vi "Map Initialization Behaviour.vi"(11 "initialize and close session behavior in":T1) -> (3 "initialization_behavior":T2)   [LabVIEW 2021, in "Session Management niDAQmx.lvlib" / "Session Factory.lvclass"]
doc: "Maps the measurement plug-in initialization behavior enum with the gRPC DAQmx initialization behaviour enum."
uses:
  Session Factory.lvclass
  NI DAQmx Client/RPC Messages/nidevice_grpc_SessionInitializationBehavior.ctl
  <vilib>/Plug-In SDKs/Sessions/Instrument/ISession Factory/Initialize and Close Session Behavior.ctl
  NI DAQmx Client/NI_DAQmx_client.lvlib
  <vilib>/Plug-In SDKs/Sessions/Instrument/ISession Factory/ISession Factory.lvclass
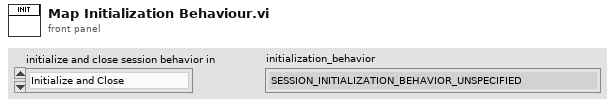
[diagram p1: front panel]
types:
  T1 = typedef "NI Session Management Instrument.lvlib/ISession Factory.lvclass/Initialize and Close Session Behavior.ctl" = enum16{"Initialize and Close", "Attach and Detach", "Initialize and Detach", "Attach and Close"}
  T2 = typedef "NI_DAQmx_client.lvlib/nidevice_grpc_SessionInitializationBehavior.ctl" = enum32{"SESSION_INITIALIZATION_BEHAVIOR_UNSPECIFIED", "SESSION_INITIALIZATION_BEHAVIOR_INITIALIZE_NEW", "SESSION_INITIALIZATION_BEHAVIOR_ATTACH_TO_EXISTING"}
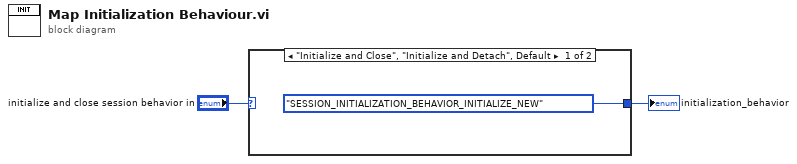
[diagram p0: block diagram]
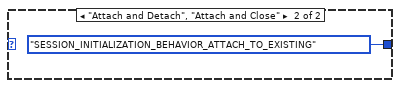
[diagram p2: hidden frame]
diagram:
  n1 = case shown="\"Initialize and Close\", \"Initialize and Detach\", Default" "initialize and close session behavior in" {
    tunnel: [nidevice_grpc_SessionInitializationBehavior."SESSION_INITIALIZATION_BEHAVIOR_INITIALIZE_NEW" ("initialization_behavior") nidevice_grpc_SessionInitializationBehavior."SESSION_INITIALIZATION_BEHAVIOR_ATTACH_TO_EXISTING" ("initialization_behavior")] -> w2
    frame "Initialize and Close", "Initialize and Detach", Default {
    }
    frame "Attach and Detach", "Attach and Close" {
    }
  }
  "initialization_behavior" <- w2
